vi "doc_delete_table.vi"(7 "table":string, 8 "error in (no error)":errorcluster, 10 "Doc in":refnum<class "Doc.lvclass">) -> (0 "error out":errorcluster, 2 "Doc out":refnum<class "Doc.lvclass">, 4 "deleted?":bool)   [LabVIEW 2020, in "toml.lvclass"]
uses:
  Doc/Doc.lvclass
  toml.lvclass
  toml.lvclass/toml.ctl
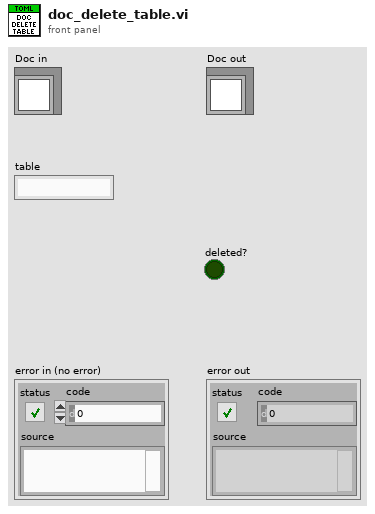
[diagram p1: front panel]
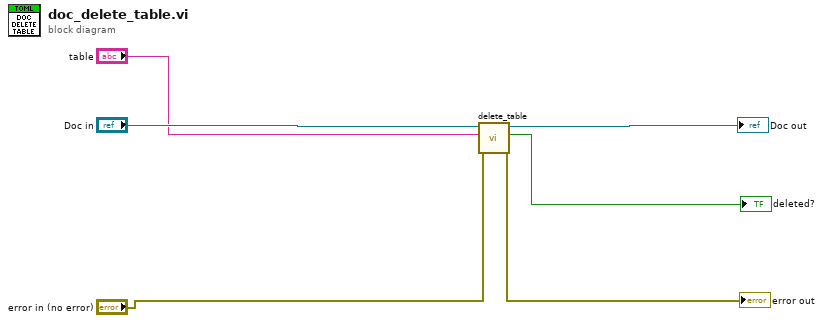
[diagram p0: block diagram]
diagram:
  n1 = call "delete_table.vi"("error in (no error)"="error in (no error)", "table_name"="table", "Doc in"="Doc in") -> ("error out"=→"error out":errorcluster, "deleted?"=→"deleted?":bool, "Doc out"=→"Doc out":refnum<class "Doc.lvclass">)  [unwired: 6 in]
